vi "Example 2 - TDMS to JMP.vi"(8 "error in (no error)":errorcluster, 11 "Path":path) -> (0 "error out":errorcluster, 2 "Array":T2(array[cluster]))   [LabVIEW 2019]
uses:
  <vilib>/Utility/Data Type/Type Definitions/Data Type.ctl
  <vilib>/Utility/Data Type/NI_Data Type.lvlib
  <instrlib>/LV_JMP_bridge/JMP Automation.lvlib
  <instrlib>/LV_JMP_bridge/DataTable/Add DataTable Variable (string).vi
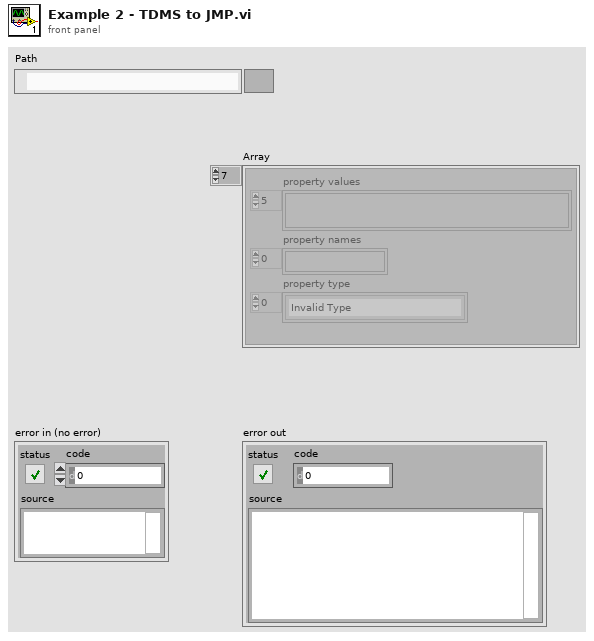
[diagram p1: front panel]
types:
  T1 = typedef "NI_Data Type.lvlib/Data Type.ctl" = enum8{"Invalid Type", "Void", "I8", "I16", "I32", "I64", "U8", "U16", "U32", "U64", "Single Float", "Double Float", "Extended Float", "Single Complex", "Double Complex", "Extended Complex", "Enum U8", "Enum U16", "Enum U32", "Enum U64", "Single Float With Unit", "Double Float With Unit", "Extended Float With Unit", "Single Complex with Unit", "Double Complex with Unit", "Extended Complex with Unit", "Boolean", "String", "Path", "Picture", "Tag", "Array", "Cluster", "Variant", "LV Variant", "Waveform", "Timestamp", "Digital Waveform", "Digital Data", "ExpressData", "Refnum", "External Data", "VI", "Poly VI", "LabVIEW Class Instance", "Fixed Point", "Set Collection", "Map Collection"}
  T2 = cluster{"property values":variant[], "property names":string[], "property type":T1[]}[]
  T3 = cluster{"property values":variant[], "property names":string[], "property type":T1[]}
  T4 = enum16{"open", "open or create", "create or replace", "create", "open (read-only)"}
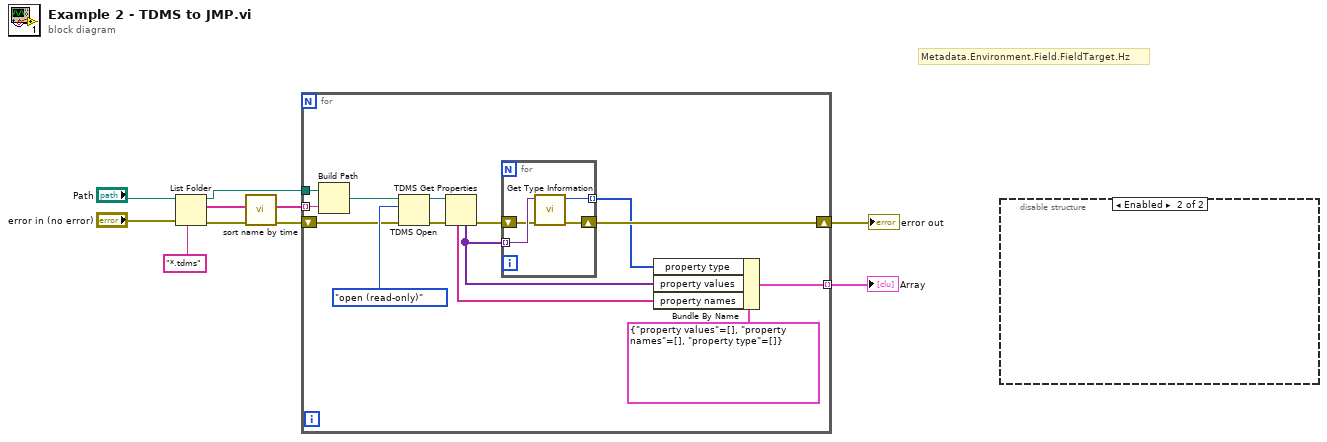
[diagram p0: block diagram]
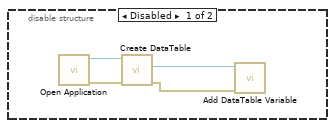
[diagram p2: hidden frame]
diagram:
  # "Metadata.Environment.Field.FieldTarget.Hz"
  n1 = List Folder(path="Path", pattern="*.tdms", error in="error in (no error)") -> (path out=w3:path, filenames=w4:string[], error out=w6:errorcluster)  [unwired: 1 in, 1 out]
  n2 = call <instrlib>:"sort name by time.vi"("error in (no error)"=w6, "filenames"=w4) -> ("error out"=w5:errorcluster, "sorted filename"=w2:string[])  [unwired: 8 in]
  n3 = for {
    shift-right: [w19] -> w8
    shift-left: w5 -> [w22]
    tunnel: [w14] -> w1 mode=indexing
    tunnel: w3 -> [w12]
    tunnel: w2 -> [w11] mode=indexing
    n4 = Build Path(base path=w12, name or relative path=w11) -> (appended path=w13:path)
    n5 = TDMS Open(8:w22, 10:T4."open (read-only)" ("operation (0:open)"), 11:w13) -> (0:w21:errorcluster, 3:w23:refnum<k34>)  [unwired: 4 in]
    n6 = TDMS Get Properties(8:w21, 11:w23) -> (0:w20:errorcluster, 4:w16:variant[], 6:w15:string[])  [unwired: 4 in, 3 out]
    n7 = for {
      tunnel: w16 -> [w28] mode=indexing
      shift-right: [w26] -> w19
      shift-left: w20 -> [w27]
      tunnel: [w25] -> w17 mode=indexing
      n8 = call <vilib>:"Get Type Information.vi"("error in (no error)"=w27, "variant"=w28) -> ("error out"=w26:errorcluster, "type"=w25:T1)  [unwired: 5 in, 3 out]
    }
    n9 = Bundle By Name(cluster=T3 {"property values"=[], "property names"=[], "property type"=[]}, "property type"=w17, "property values"=w16, "property names"=w15) -> (w14:T3)
  }
  "error out" <- w8
  "Array" <- w1
  n10 = disable-structure shown="Enabled" {
    frame Disabled {
      n11 = call <instrlib>:"Open Application.vi"() -> ("error out"=w30:errorcluster, "JMP application"=w31:refnum<k7>)  [unwired: 10 in]
      n12 = call <instrlib>:"Create DataTable.vi"("error in (no error)"=w30, "JMP application"=w31) -> ("error out"=w29:errorcluster, "new DataTable"=w32:refnum<k7>)  [unwired: 7 in, 1 out]
      n13 = call-poly <instrlib>:"Add DataTable Variable.vi"("error in (no error)"=w29, "JMP DataTable"=w32) -> ()  [unwired: 8 in, 2 out]
    }
    frame Enabled {
    }
  }
